vi "10-4 Create Table.vi"() -> ()   [LabVIEW 2014]
uses:
  <vilib>/addons/database/Auxilliary.llb/DB Tools Column Info.ctl
  <vilib>/addons/database/Auxilliary.llb/DB Tools DataTypes.ctl
  <vilib>/addons/database/Connection.llb/DB Tools Open Connec (Path).vi
  <vilib>/addons/database/NI_Database_API.lvlib
panel:
  in  "connection information":path
  out "error out":errorcluster
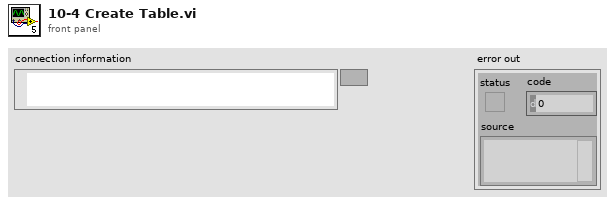
[diagram p1: front panel]
types:
  T1 = typedef "NI_Database_API.lvlib/DB Tools Column Info.ctl" = cluster{"column name":string, "data type":T2, "size":i32, "allow null?":bool}
  T2 = typedef "NI_Database_API.lvlib/DB Tools DataTypes.ctl" = enum16{"String", "Long (I32)", "Single (SGL)", "Double (DBL)", "Date/Time", "Binary"}
  T3 = typedef "NI_Database_API.lvlib/Conn ObjectReference.ctl" = refnum<k1>
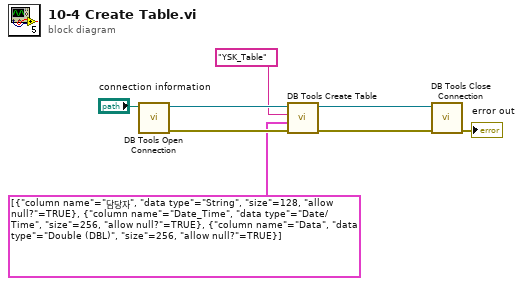
[diagram p0: block diagram]
diagram:
  n1 = call-poly <vilib>:"DB Tools Open Connection.vi"("connection information"="connection information") -> ("error out"=w5:errorcluster, "connection reference"=w8:T3)  [unwired: 7 in]
  n2 = call <vilib>:"DB Tools Create Table.vi"("error in (no error)"=w5, "column information"=T1[] [{"column name"="담당자", "data type"=enum."String", "size"=128, "allow null?"=TRUE}, {"column name"="Date_Time", "data type"=enum."Date/Time", "size"=256, "allow null?"=TRUE}, {"column name"="Data", "data type"=enum."Double (DBL)", "size"=256, "allow null?"=TRUE}], "table"="YSK_Table", "connection reference"=w8) -> ("error out"=w6:errorcluster, "connection reference out"=w7:T3)  [unwired: 4 in]
  n3 = call <vilib>:"DB Tools Close Connection.vi"("error in (no error)"=w6, "connection reference"=w7) -> ("error out"=→"error out":errorcluster)  [unwired: 5 in]
